vi "Generate Warning.vi"(8 "error in":errorcluster, 10 "Warning":cluster{"Warning Text":string, "code":i32}={"Warning Text"="", "code"=5000008}, 11 "Instruments in":refnum<class "Instruments.lvclass">) -> (0 "error out":errorcluster, 3 "Instruments out":refnum<class "Instruments.lvclass">)   [LabVIEW 2023, in "Instruments.lvlib" / "Instruments.lvclass"]
uses:
  Library/Instruments.lvclass
  C:/Users/Public/Documents/Development/builds/Engine/Actor Framework.lvlibp/1abvi3w/vi.lib/ActorFramework/Actor/Actor.lvclass
  builds/Engine/Actor Framework.lvlibp/1abvi3w/vi.lib/ActorFramework/Actor/Read Actor Label.vi
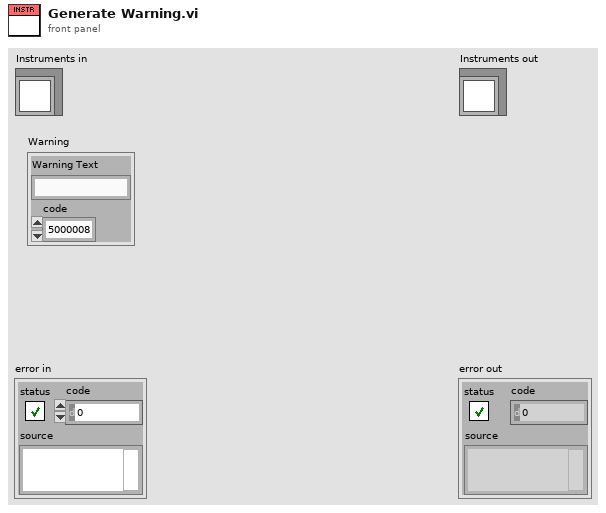
[diagram p1: front panel]
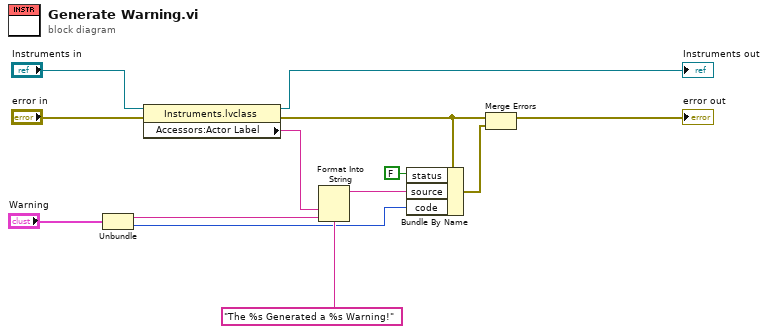
[diagram p0: block diagram]
diagram:
  n1 = Unbundle("Warning") -> ("Warning Text"=w2:string, "code"=w1:i32)
  n2 = property class="Instruments.lvclass"(reference="Instruments in", error in="error in") -> (reference out=→"Instruments out":refnum<class "Instruments.lvclass">, error out=w10:errorcluster, "Accessors:Actor Label"=w12:string)
  n3 = Format Into String(format string="The %s Generated a %s Warning!", w12, w2) -> (resulting string=w7:string)  [unwired: 2 in, 1 out]
  n4 = Bundle By Name(cluster=w10, "status"=FALSE, "source"=w7, "code"=w1) -> (w9:errorcluster)
  n5 = Merge Errors(w10, w9) -> (→"error out":errorcluster)
